vi "SVFA Peak Amplitude and Relative Phase.vi"   [LabVIEW 2017]
doc: "Use this VI to compute FFT spectra with magnitude equal to response magnitude and phase equal to response relative to reference. Use the N responses, 1 stimulus instance to compute phase-assigned auto spectra for multiple response channels."
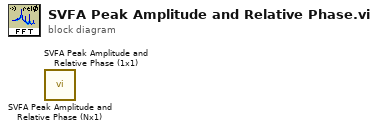
[diagram p0: block diagram]
diagram:
  n1 = call <vilib>:"SVFA Peak Amplitude and Relative Phase (Nx1).vi"() -> ()  [unwired: 11 in, 9 out]
  n2 = call <vilib>:"SVFA Peak Amplitude and Relative Phase (1x1).vi"() -> ()  [unwired: 11 in, 9 out]
